vi "CreateNewProperty.vi"(7 "Property In":T3, 8 "error in":errorcluster, 9 "Comm  In":T2, 11 "Device In":T1={"Name"="", "BaseURL"="", "AppKey"="", "Headers"=["Content-Type:application/json"], "Timeout"=10000, "Identifier"="", "Password"="", "Comments"="", "Handle"=0, "# Handles"=0}) -> (0 "error out":errorcluster, 1 "Comm Out":T2, 3 "Device Out":T1={"Name"="", "BaseURL"="", "AppKey"="", "Headers"=["Content-Type:application/json"], "Timeout"=10000, "Identifier"="", "Password"="", "Comments"="", "Handle"=0, "# Handles"=0})   [LabVIEW 2016]
uses:
  _subVIs/HTTPComm.ctl
  _subVIs/Device.ctl
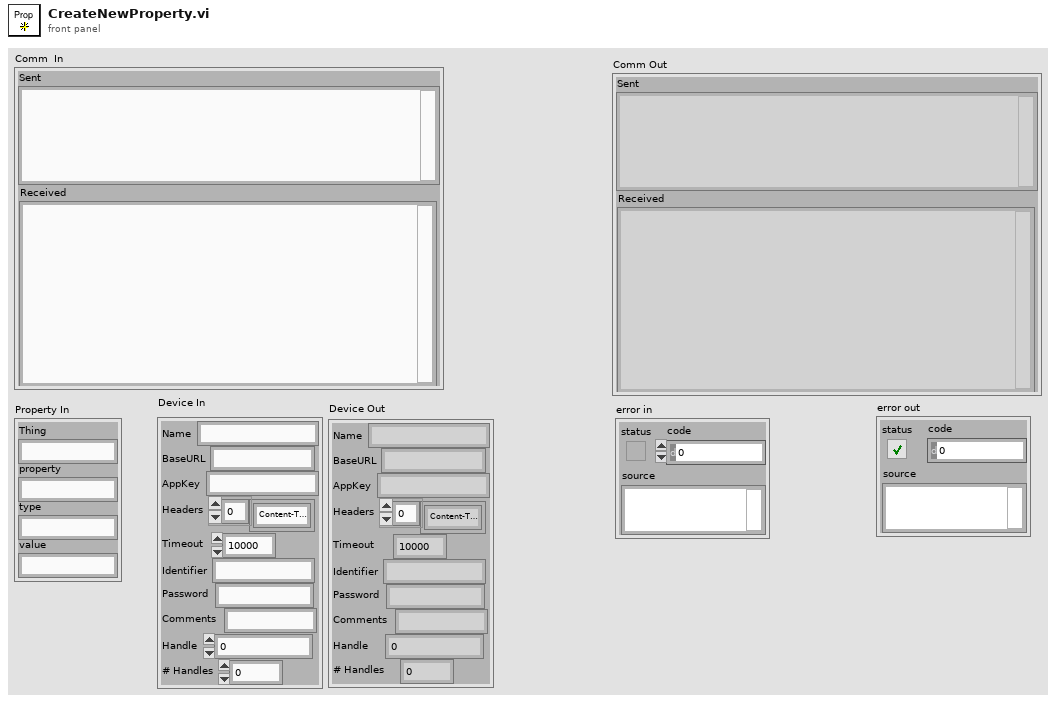
[diagram p1: front panel]
types:
  T1 = typedef "Device.ctl" = cluster{"Name":string, "BaseURL":string, "AppKey":string, "Headers":string[], "Timeout":i32, "Identifier":string, "Password":string, "Comments":string, "Handle":u32, "# Handles":i32}
  T2 = typedef "HTTPComm.ctl" = cluster{"url":string, "sent headers":string, "sent body":string, "headers":string, "body":string, "Sent":string, "Received":string}
  T3 = cluster{"Thing":string, "property":string, "type":string, "value":string}
  T4 = cluster{"name":string, "type":string, "logged":bool}
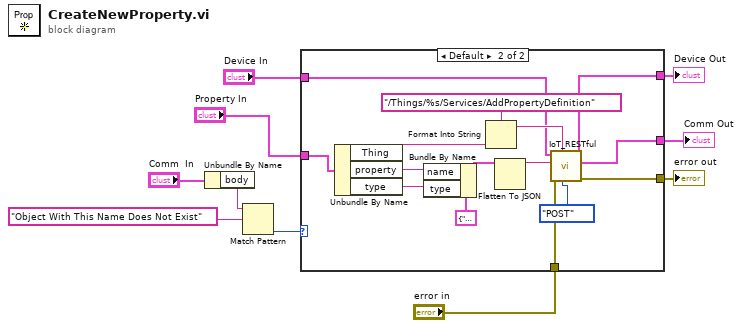
[diagram p0: block diagram]
diagram:
  n1 = Unbundle By Name("Comm  In") -> ("body"=w8:string)
  n2 = Match Pattern(string=w8, regular expression="Object With This Name Does Not Exist") -> (offset past match=w9:i32)  [unwired: 1 in, 3 out]
  n3 = case shown="Default" w9 {
    tunnel: "Property In" -> [_ w25]
    tunnel: "error in" -> [w11 w18]
    tunnel: [w11 w17] -> w4
    tunnel: "Device In" -> [w12 w16]
    tunnel: [w12 w15] -> w2
    tunnel: [_ w14] -> w1
    frame -1 {
    }
    frame Default {
      n4 = Unbundle By Name(w25) -> ("Thing"=w24:string, "property"=w22:string, "type"=w21:string)
      n5 = Bundle By Name(cluster=T4 {"name"="", "type"="", "logged"=FALSE} ("Property"), "name"=w22, "type"=w21) -> (w20:T4)
      n6 = Format Into String(format string="/Things/%s/Services/AddPropertyDefinition", w24) -> (resulting string=w23:string)  [unwired: 2 in, 1 out]
      n7 = Flatten To JSON(anything=w20) -> (JSON string=w19:string)  [unwired: 2 in, 1 out]
      n8 = call "IoT_RESTful.vi"("Method"=enum16{"GET", "PUT", "POST", "MultiPOST"}."POST", "url"=w23, "error in"=w18, "JSON"=w19, "Device In"=w16) -> ("error out"=w17:errorcluster, "Comm"=w14:T2, "Device Out"=w15:T1)  [unwired: 3 in, 1 out]
    }
  }
  "error out" <- w4
  "Comm Out" <- w1
  "Device Out" <- w2
